vi "get camera driver.vi"(8 "error in (no error)":errorcluster, 9 "Path":path, 10 "Section":string, 11 "Imaq Camera Driver Factroy in":refnum<class "Imaq Camera Driver Factory.lvclass">) -> (0 "error out":errorcluster, 2 "Camera Driver.lvclass":refnum<class "Camera Driver.lvclass">, 3 "Imaq Camera Driver Factroy out":refnum<class "Imaq Camera Driver Factory.lvclass">)   [LabVIEW 2022 SP3, in "Imaq Camera Driver Factory.lvclass"]
uses:
  Imaq Camera Driver Factory.lvclass
  Camera Driver/Camera Driver.lvclass
  Imaq Camera Driver Factory.lvclass/Imaq Camera Driver Factory.ctl
  imaq camera driver/Imaq Camera.lvclass
  C:/XY Stage/Camera/imaq camera driver/Imaq Camera.lvclass
  C:/XY Stage/Camera/Camera Driver/Camera Driver.lvclass
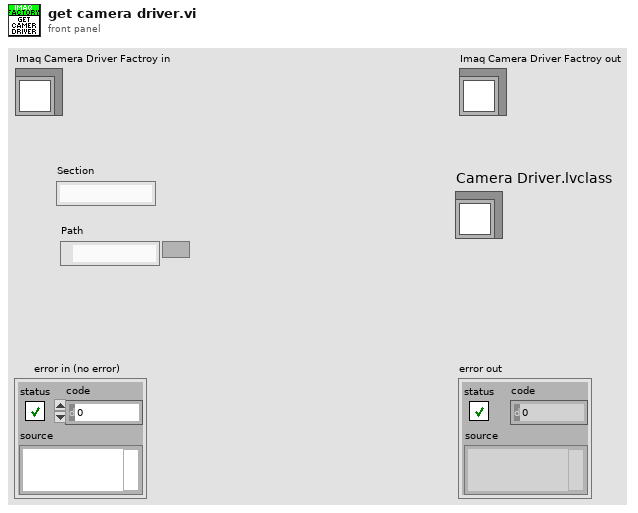
[diagram p1: front panel]
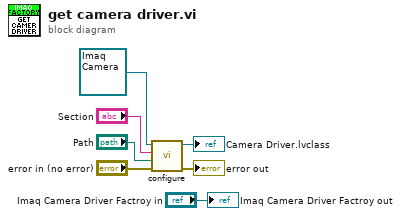
[diagram p0: block diagram]
diagram:
  n1 = call "configure.vi"("error in (no error)"="error in (no error)", "Path"="Path", "Section"="Section", "Imaq Camera in"=refnum<class "Imaq Camera.lvclass"> refnum ("Imaq Camera.lvclass")) -> ("error out"=→"error out":errorcluster, "Imaq Camera out"=→"Camera Driver.lvclass":refnum<class "Imaq Camera.lvclass">)  [unwired: 6 in]
  "Imaq Camera Driver Factroy out" <- "Imaq Camera Driver Factroy in"
